vi "Lab1_Exercise3.vi"() -> ()   [LabVIEW 2016]
panel:
  in  "Enum":T1(ring)
  in  "Numeric 2":dbl
  in  "Number 1":dbl
  out "Result":dbl
  out "Error LED":bool
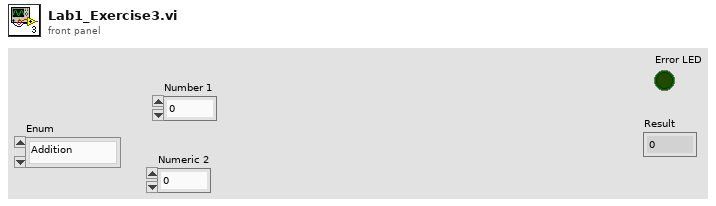
[diagram p1: front panel]
types:
  T1 = enum16{"Addition", "Subtraction", "Multiplication", "Division"}
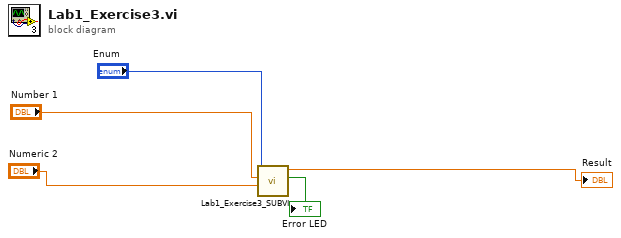
[diagram p0: block diagram]
diagram:
  n1 = call "Lab1_Exercise3_SUBVI.vi"("Numeric in"="Numeric 2", "Number 1"="Number 1", "Enum"="Enum") -> ("Error LED"=→"Error LED":bool, "Numeric out"=→"Result":dbl)  [unwired: 7 in]
